vi "PlotsDadosBrutos.vi"(1 "Pasta do ensaio":path=path "L:/Documentos/Serviços já concluidos/Tensão residual/Molas Volvo/Dados/Terceiro grupo/Amostra_1_0", 2 "Pasta das imagens":path=path "L:/Documentos/Serviços já concluidos/Tensão residual/Molas Volvo/Dados/Terceiro grupo/Amostra_1_0") -> ()   [LabVIEW 2016]
panel:
  out "Deformações":dbl[][](graph)
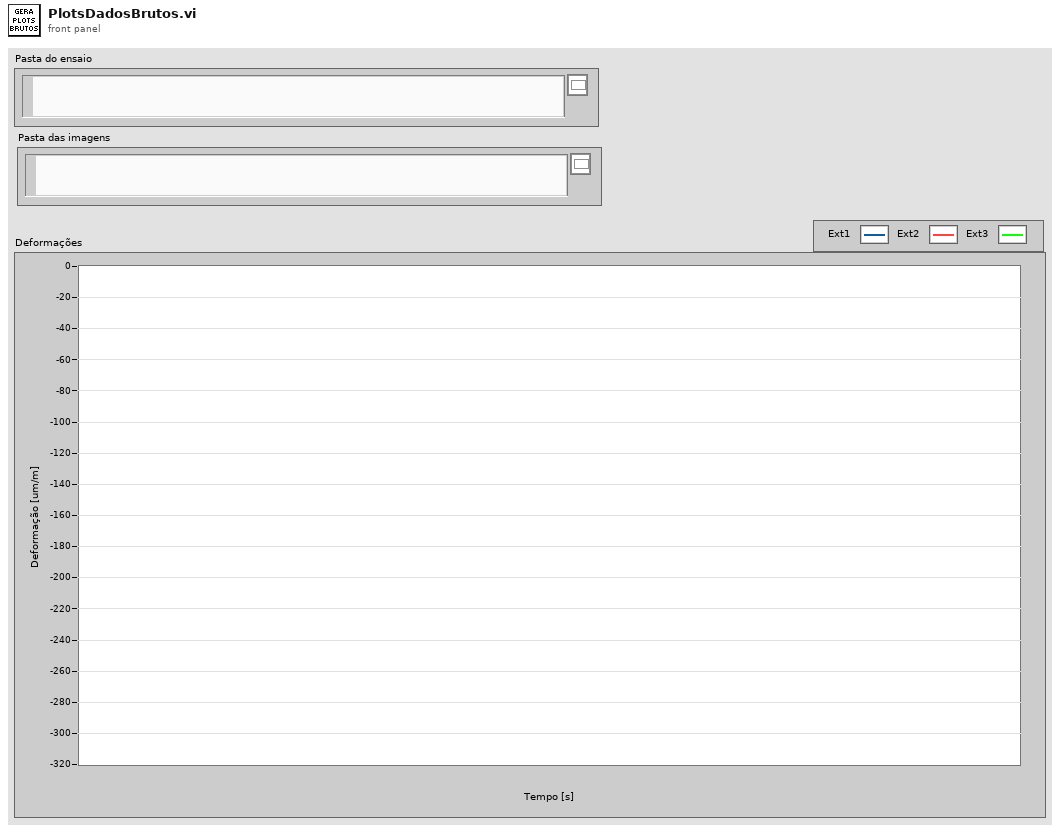
[diagram p1: front panel]
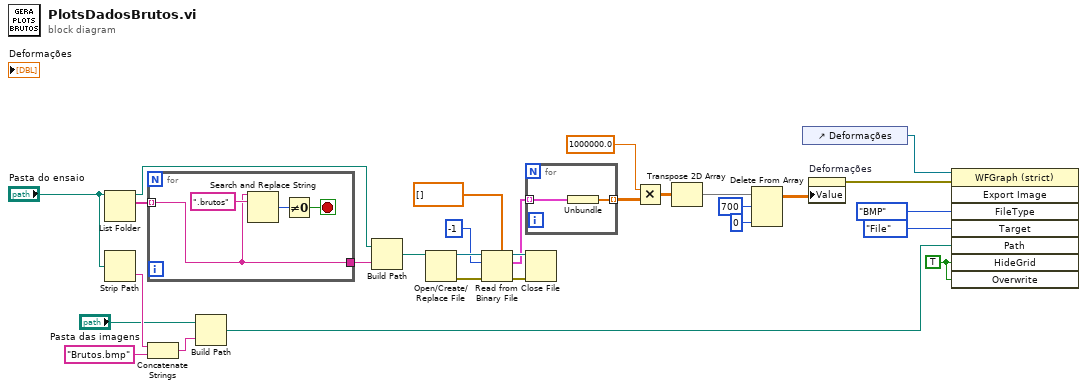
[diagram p0: block diagram]
diagram:
  w9 = TRUE ("Hide Grid")
  n1 = List Folder(path="Pasta do ensaio") -> (path out=w28:path, filenames=w20:string[])  [unwired: 3 in, 2 out]
  n2 = Strip Path(path="Pasta do ensaio") -> (name=w14:string)  [unwired: 1 out]
  n3 = for {
    tunnel: w20 -> [w30] mode=indexing
    tunnel: [w30] -> w29
    stop <- w31 stop-if-true
    n4 = Search and Replace String(input string=w30, search string=".brutos" ("replace string (\"\")")) -> (number of replacements=w32:i32)  [unwired: 6 in, 3 out]
    n5 = Not Equal To 0?(x=w32) -> (x != 0?=w31:bool)
  }
  n6 = Concatenate Strings(w14, "Brutos.bmp" ("string")) -> (w11:string)
  n7 = Build Path(base path="Pasta das imagens", name or relative path=w11) -> (appended path=w10:path)
  n8 = Build Path(base path=w28, name or relative path=w29) -> (appended path=w27:path)
  n9 = Open/Create/Replace File(file path (use dialog)=w27) -> (refnum out=w26:refnum<file>, error out=w23:errorcluster)  [unwired: 5 in, 1 out]
  n10 = Read from Binary File(5:dbl[] [], 8:w23, 10:-1 ("count (1)"), 11:w26) -> (0:w22:errorcluster, 2:w19:cluster{dbl[]}[], 3:w21:refnum<file>)  [unwired: 2 in, 1 out]
  n11 = for {
    tunnel: w19 -> [w35] mode=indexing
    tunnel: [w34] -> w7 mode=indexing
    n12 = Unbundle(w35) -> (w34:dbl[])
  }
  n13 = Close File(refnum=w21, error in=w22) -> ()  [unwired: 2 out]
  n14 = Multiply(x=1000000.0, y=w7) -> (x*y=w5:dbl[][])
  n15 = Transpose 2D Array(2D array=w5) -> (transposed array=w4:dbl[][])
  n16 = Delete From Array(array=w4, length=700, index (col)=0 ("disabled index (col)")) -> (array with subset deleted=w3:dbl[][])  [unwired: 1 in, 1 out]
  n17 = control-ref of="Deformações"() -> (w16:refnum<vi>)
  n18 = property on="Deformações" class="WFGraph (strict)"("Value"=w3) -> (error out=w8:errorcluster)  [unwired: 2 in, 1 out]
  n19 = invoke class="WFGraph (strict)" method="Export Image"(reference=w16, error in=w8, "FileType"=enum32{"BMP", "EPS", "EMF", "PICT"}."BMP" ("File Type"), "Target"=enum32{"File", "Clipboard"}."File", "Path"=w10, "HideGrid"=w9, "Overwrite"=w9) -> ()  [unwired: 1 in, 8 out]
